vi "Feature_Names.vi"(8 "error in (no error)":errorcluster caption="entrée d'erreur (pas d'erreur)", 11 "Load_Diabetes en entrée":refnum<class "Load_Diabetes.lvclass">) -> (0 "error out":errorcluster caption="sortie d'erreur", 3 "Load_Diabetes en sortie":refnum<class "Load_Diabetes.lvclass">)   [LabVIEW 2020, in "Load_Diabetes.lvclass"]
uses:
  Load_Diabetes.lvclass
  Load_Diabetes.lvclass/Load_Diabetes.ctl
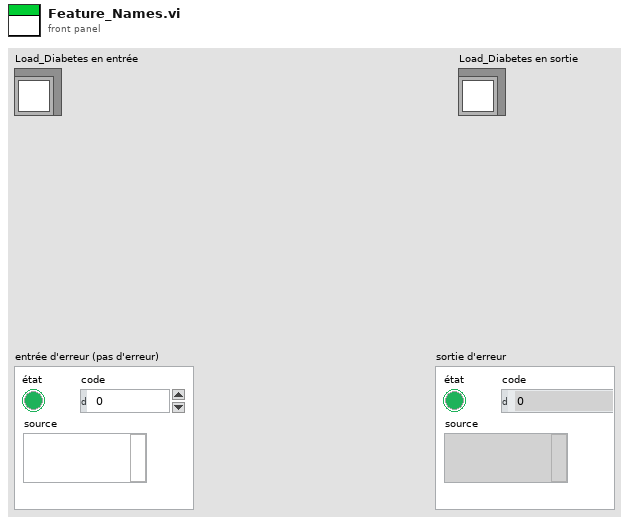
[diagram p1: front panel]
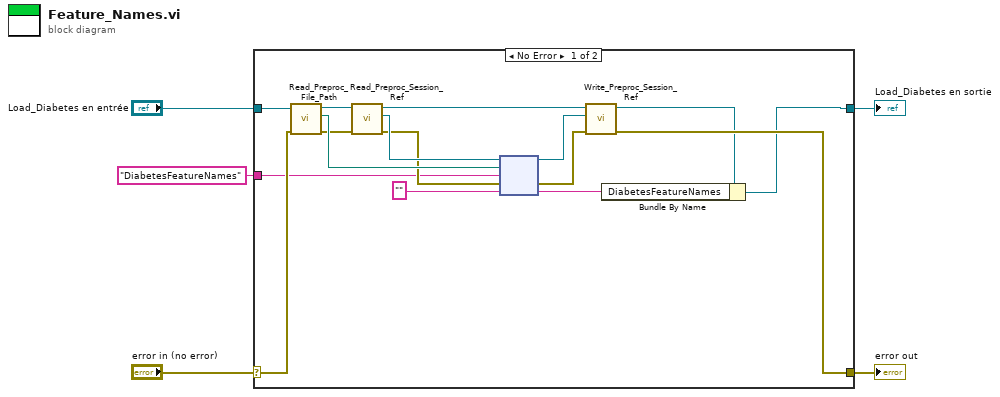
[diagram p0: block diagram]
diagram:
  n1 = case shown="No Error" "error in (no error)" {
    selector: "error in (no error)" -> [w11 w23]
    tunnel: [w10 w23] -> w4
    tunnel: [w8 w22] -> w2
    tunnel: "Load_Diabetes en entrée" -> [w9 w22]
    tunnel: "DiabetesFeatureNames" -> [w7 _]
    frame No Error {
      n2 = call-dynamic "Read_Preproc_File_Path.vi"("error in (no error)"=w11, "Python in"=w9) -> ("error out"=w16:errorcluster, "File_Path"=w19:path, "Python out"=w21:refnum<class "Load_Diabetes.lvclass">)  [unwired: 7 in]
      n3 = call-dynamic "Read_Preproc_Session_Ref.vi"("error in (no error)"=w16, "Python in"=w21) -> ("error out"=w17:errorcluster, "Session_ref"=w18:refnum<k35>, "Python out"=w20:refnum<class "Load_Diabetes.lvclass">)  [unwired: 7 in]
      n4 = node(w18, w19, w7, w17, "") -> (w13:refnum<k35>, w15:errorcluster, w12:string)  [unwired: 2 out]
      n5 = call-dynamic "Write_Preproc_Session_Ref.vi"("error in (no error)"=w15, "Session_ref"=w13, "Python in"=w20) -> ("error out"=w10:errorcluster, "Python out"=w6:refnum<class "Load_Diabetes.lvclass">)  [unwired: 7 in]
      n6 = Bundle By Name(cluster=w6, "DiabetesFeatureNames"=w12) -> (w8:refnum<class "Load_Diabetes.lvclass">)
    }
    frame Error {
    }
  }
  "error out" <- w4
  "Load_Diabetes en sortie" <- w2
